vi "Práctica01_Ejercicio3_1.vi"() -> ()   [LabVIEW 2020]
uses:
  <vilib>/numeric/Random Number (Range) DBL.vi
panel:
  out "Waveform Graph":dynamicdata(graph)
  out "Filtro EMA":dbl[](array[numeric])
  out "Centigrados-Or":dbl[](array[numeric])
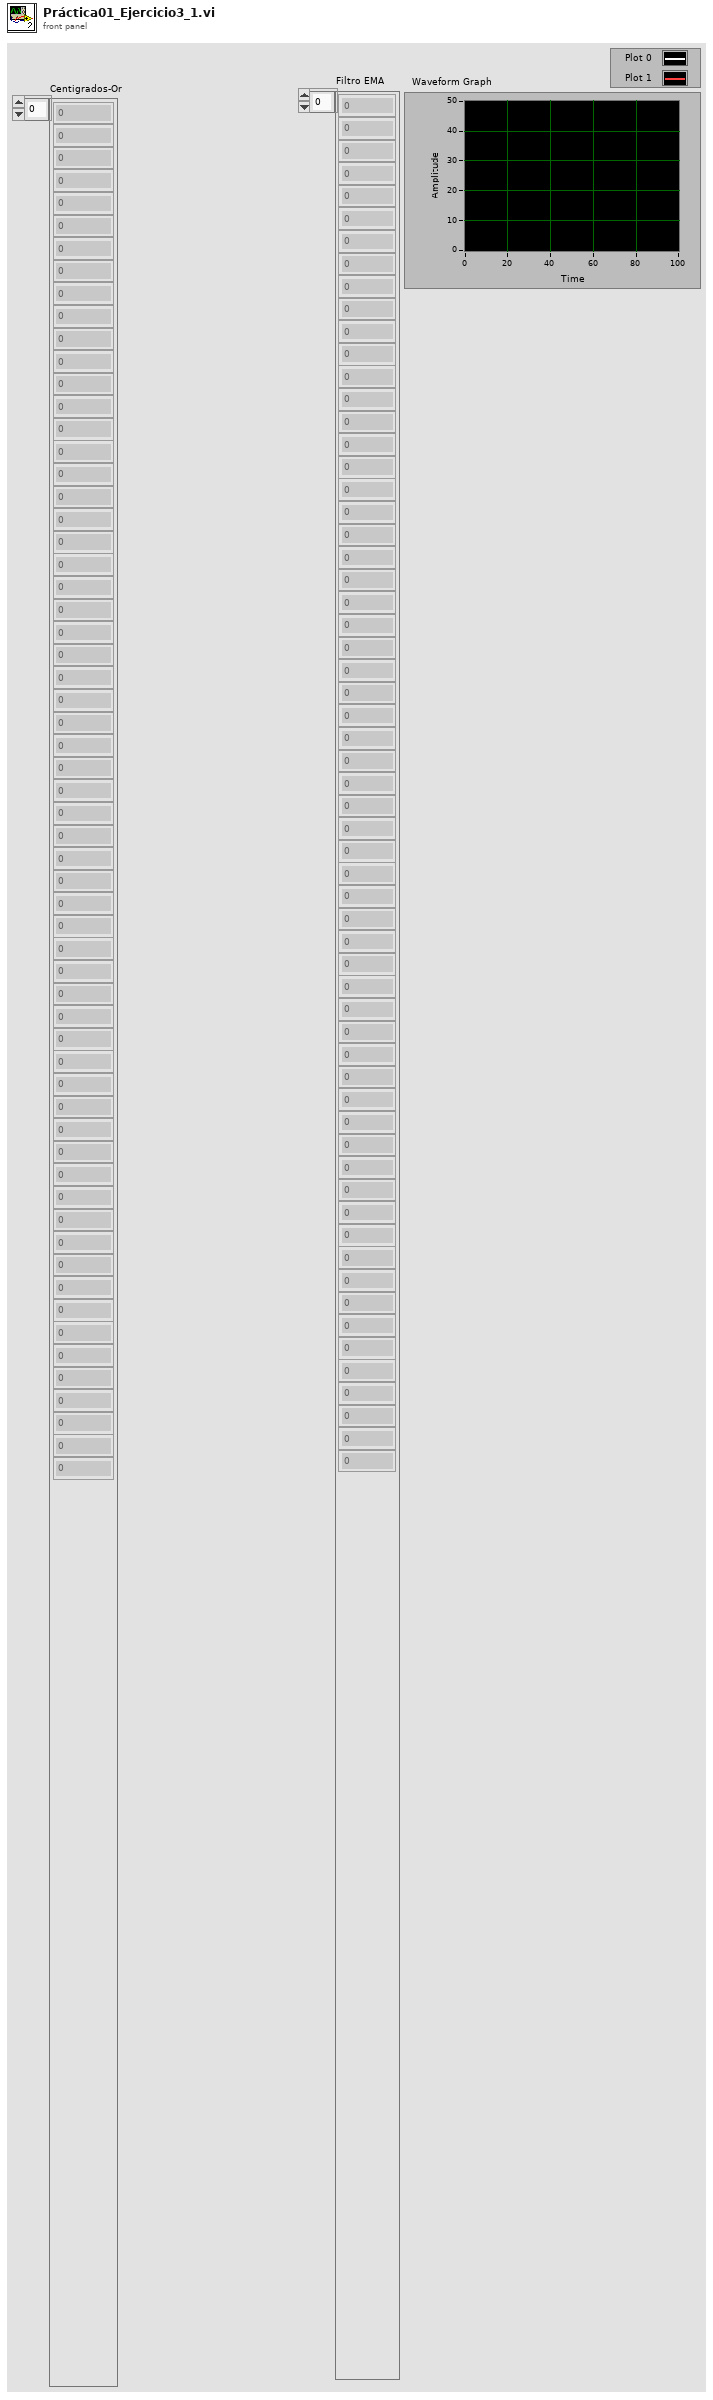
[diagram p1: front panel]
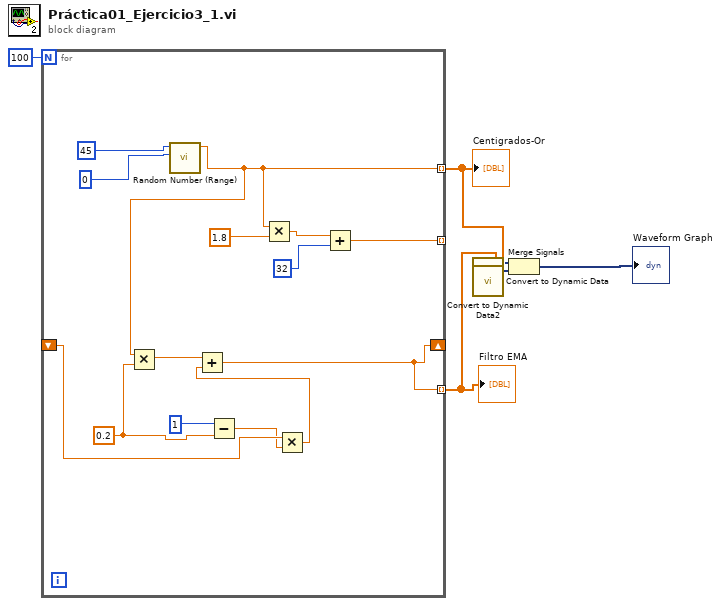
[diagram p0: block diagram]
diagram:
  n1 = for {
    N: 100 -> [_]
    tunnel: [w11] -> w3 mode=indexing
    tunnel: [w15] -> _ mode=indexing
    shift-right: [w7] -> _
    shift-left: _ -> [w9]
    tunnel: [w7] -> w5 mode=indexing
    w12 = 0.2
    n2 = call-poly <vilib>:"Random Number (Range).vi"("lower bound (0)"=0, "upper bound (100)"=45) -> ("number"=w11:dbl)  [unwired: 9 in]
    n3 = Multiply(x=w11, y=w12) -> (x*y=w14:dbl)
    n4 = Subtract(x=1, y=w12) -> (x-y=w8:dbl)
    n5 = Multiply(x=w11, y=1.8) -> (x*y=w16:dbl)
    n6 = Multiply(x=w9, y=w8) -> (x*y=w10:dbl)
    n7 = Add(x=w14, y=w10) -> (x+y=w7:dbl)
    n8 = Add(x=w16, y=32) -> (x+y=w15:dbl)
  }
  "Centigrados-Or" <- w3
  "Filtro EMA" <- w5
  n9 = call "Convert to Dynamic Data2"("Array"=w3) -> ("Dynamic Data Type"=w2:dynamicdata)  [unwired: 3 in]
  n10 = call "Convert to Dynamic Data"("Array"=w5) -> ("Dynamic Data Type"=w4:dynamicdata)  [unwired: 3 in]
  n11 = Merge Signals(w2, w4) -> (→"Waveform Graph":dynamicdata)
